vi "configure_standar_waveform (SubVI).vi"(4 "DC Offset (0 V)":i8, 6 "Frequency (1000 Hz)":i16=127, 7 "Waveform Function (0: Sine) in":u16(ring) items=["Sine", "Square", "Ramp", "Pulse", "Noise", "DC "], 8 "error in (no error)":errorcluster, 9 "Amplitude (5.0 Vpp)":i8=5, 10 "Phase":i16(knob) scale=0.0..360.0, 11 "VISA Refnum in":refnum<visa-resource-name>) -> (0 "error out":errorcluster, 3 "VISA Refnum out":refnum<visa-resource-name>)   [LabVIEW 2023]
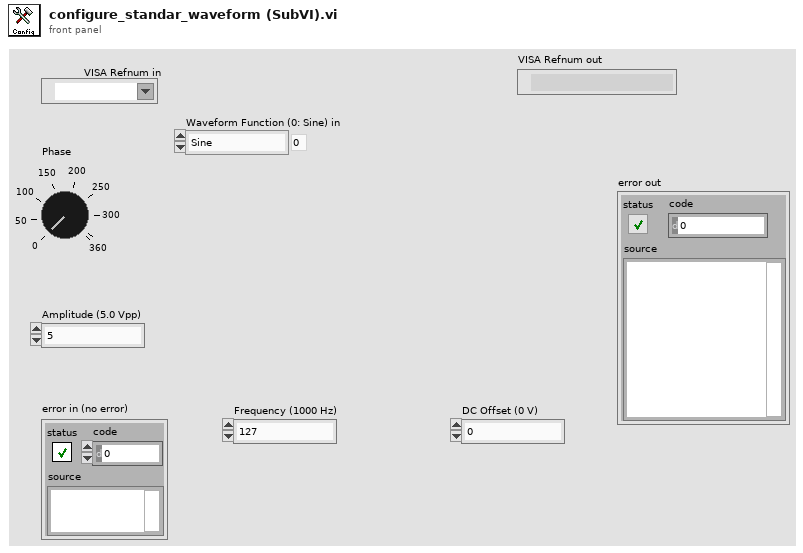
[diagram p1: front panel]
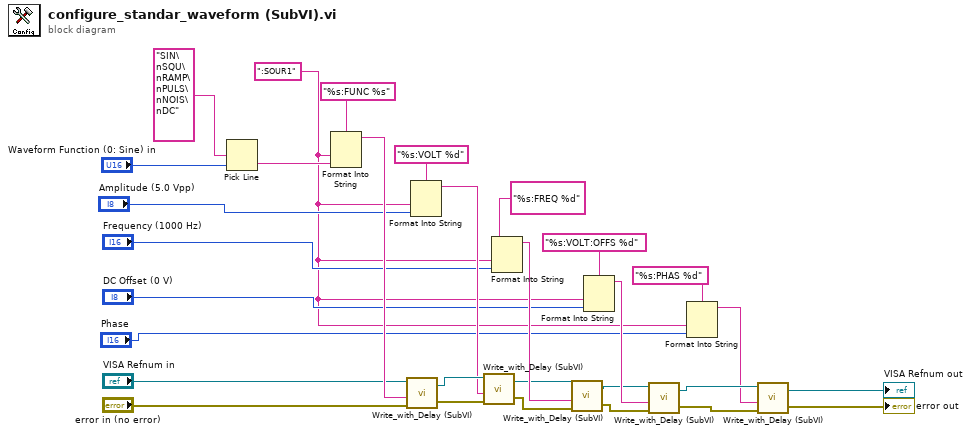
[diagram p0: block diagram]
diagram:
  w4 = ":SOUR1"
  n1 = Pick Line(multi-line string="SIN\nSQU\nRAMP\nPULS\nNOIS\nDC" ("string (\"\")"), line index="Waveform Function (0: Sine) in") -> (output string=w12:string)  [unwired: 1 out]
  n2 = Format Into String(format string="%s:FUNC %s", w4, w12) -> (resulting string=w17:string)  [unwired: 2 in, 1 out]
  n3 = call "Write_with_Delay (SubVI).vi"("error in (no error)"="error in (no error)", "Command"=w17, "VISA Refnum in"="VISA Refnum in") -> ("error out"=w19:errorcluster, "VISA Refnum out"=w21:refnum<visa-resource-name>)  [unwired: 1 in]
  n4 = Format Into String(format string="%s:VOLT %d", w4, "Amplitude (5.0 Vpp)") -> (resulting string=w20:string)  [unwired: 2 in, 1 out]
  n5 = call "Write_with_Delay (SubVI).vi"("error in (no error)"=w19, "Command"=w20, "VISA Refnum in"=w21) -> ("error out"=w27:errorcluster, "VISA Refnum out"=w22:refnum<visa-resource-name>)  [unwired: 1 in]
  n6 = Format Into String(format string="%s:FREQ %d", w4, "Frequency (1000 Hz)") -> (resulting string=w24:string)  [unwired: 2 in, 1 out]
  n7 = call "Write_with_Delay (SubVI).vi"("error in (no error)"=w27, "Command"=w24, "VISA Refnum in"=w22) -> ("error out"=w26:errorcluster, "VISA Refnum out"=w23:refnum<visa-resource-name>)  [unwired: 1 in]
  n8 = Format Into String(format string="%s:VOLT:OFFS %d", w4, "DC Offset (0 V)") -> (resulting string=w25:string)  [unwired: 2 in, 1 out]
  n9 = call "Write_with_Delay (SubVI).vi"("error in (no error)"=w26, "Command"=w25, "VISA Refnum in"=w23) -> ("error out"=w30:errorcluster, "VISA Refnum out"=w29:refnum<visa-resource-name>)  [unwired: 1 in]
  n10 = Format Into String(format string="%s:PHAS %d", w4, "Phase") -> (resulting string=w28:string)  [unwired: 2 in, 1 out]
  n11 = call "Write_with_Delay (SubVI).vi"("error in (no error)"=w30, "Command"=w28, "VISA Refnum in"=w29) -> ("error out"=→"error out":errorcluster, "VISA Refnum out"=→"VISA Refnum out":refnum<visa-resource-name>)  [unwired: 1 in]
